vi "MoveToRecycleBin.vi"(0 "Item Refnum":refnum<vi>, 11 "error in":errorcluster) -> (15 "error out":errorcluster)   [LabVIEW 2020]
doc: "Move the file to the recylebin\n\nCreated by Bas v. Etten 2024"
uses:
  Microsoft.VisualBasic
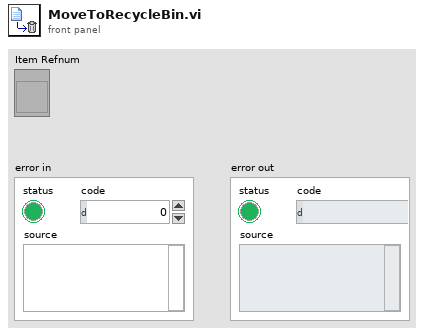
[diagram p1: front panel]
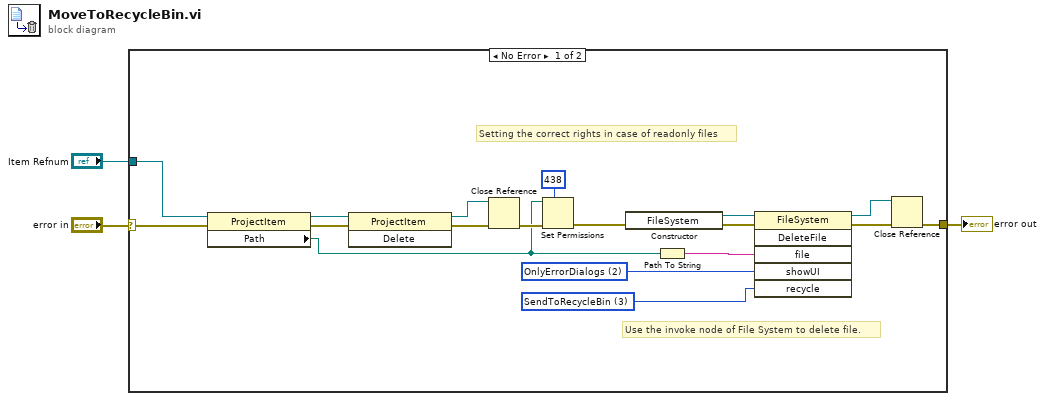
[diagram p0: block diagram]
diagram:
  n1 = case shown="No Error" "error in" {
    selector: "error in" -> [w4 w22]
    tunnel: "Item Refnum" -> [w14 _]
    tunnel: [w5 w22] -> w2
    frame No Error {
      w15 = 3 items=["DeletePermanently"=2, "SendToRecycleBin"=3] ("Delete Options")
      w16 = 2 items=["OnlyErrorDialogs"=2, "AllDialogs"=3] ("Dialog Options")
      # "Setting the correct rights in case of readonly files"
      # "Use the invoke node of File System to delete file."
      n2 = property class="ProjectItem"(reference=w14, error in=w4) -> (reference out=w11:refnum<vi>, error out=w9:errorcluster, "Path"=w7:path)
      n3 = invoke class="ProjectItem" method="Delete"(reference=w11, error in=w9) -> (reference out=w13:refnum<vi>, error out=w12:errorcluster)  [unwired: 1 in, 1 out]
      n4 = Close Reference(reference=w13, error in (no error)=w12) -> (error out=w8:errorcluster)
      n5 = Set Permissions(7:i16 438 ("permissions"), 8:w8, 11:w7) -> (0:w6:errorcluster)  [unwired: 2 in, 1 out]
      n6 = constructor class="FileSystem"(error in=w6) -> (reference out=w20:refnum<k24>, error out=w21:errorcluster)  [unwired: 2 in, 1 out]
      n7 = Path To String(path=w7) -> (string=w17:string)
      n8 = invoke class="FileSystem" method="DeleteFile"(reference=w20, error in=w21, "file"=w17, "showUI"=w16, "recycle"=w15) -> (reference out=w19:refnum<k24>, error out=w18:errorcluster)  [unwired: 1 in, 4 out]
      n9 = Close Reference(reference=w19, error in (no error)=w18) -> (error out=w5:errorcluster)
    }
    frame Error {
    }
  }
  "error out" <- w2
